vi "niFpgaFrictionTemplate.vi"(0 "gain":fxp<+/-,16,8>, 5 "input":fxp<+/-,16,16>, 9 "offset":fxp<+/-,16,16>) -> (4 "output":fxp<+/-,16,16>)   [LabVIEW 2017]
doc: "Implements a discontinuity at zero with linear behavior elsewhere. The data type you wire to <B>input</B> determines the <B>output</B> data type."
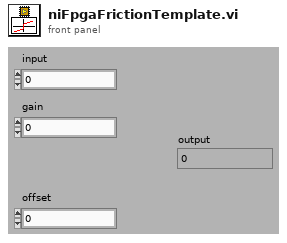
[diagram p1: front panel]
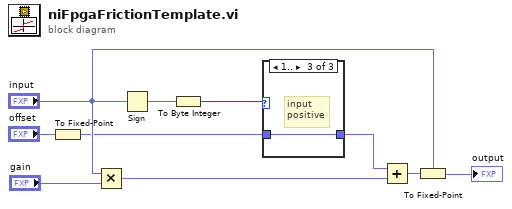
[diagram p0: block diagram]
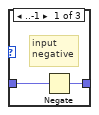
[diagram p2: hidden frame]
diagram:
  n1 = To Fixed-Point(number="offset") -> (fixed-point=w1:fxp<+/-,16,16>)  [unwired: 1 in]
  n2 = Multiply(x="input", y="gain") -> (x*y=w6:fxp<+/-,32,24>)
  n3 = Sign(1:"input") -> (0:w8:fxp<+/-,2,2>)
  n4 = To Byte Integer(number=w8) -> (8bit integer=w7:i8)
  n5 = case shown="1.." w7 {
    tunnel: w1 -> [w12 _ w13]
    tunnel: [w11 _ w13] -> w10
    frame ..-1 {
      # "input\nnegative"
      n6 = Negate(x=w12) -> (-x=w11:fxp<+/-,17,17>)
    }
    frame 0 {
      # "input\nzero"
    }
    frame 1.. {
      # "input \npositive"
    }
  }
  n7 = Add(x=w10, y=w6) -> (x+y=w9:fxp<+/-,32,24>)
  n8 = To Fixed-Point(fixed-point type="input", number=w9) -> (fixed-point=→"output":fxp<+/-,16,16>)
